vi "DCfgGlbs.vi"() -> ()   [LabVIEW 2011]
panel:
  out "Special[]":i32[](array[numeric])
  in  "Condition":i8[](array[numeric])=[0, 0, 0, 0, 0, 0, 0, 0, 0, 0, 0, 0, 0, 0, 0, 0, 0, 0, 1, 1, 1, 0, 0, 0, 0, 0, 0, 0, -9, 0]
  out "Warning[]":i32[](array[numeric])
  in  "Shutdown[]":i32[](array[numeric])=[5, 9, 11, 12, 20, 21, 22, 28, 29, 30, 31]
  out "Safe[]":i32[](array[numeric])=[0, 6, 8, 13, 14, 15, 16, 27]
  out "Din #":i32
  in  "Din Logic":bool[](array[boolean])=[TRUE, TRUE, TRUE, TRUE, FALSE, FALSE, FALSE, FALSE, TRUE, FALSE, FALSE, FALSE, FALSE, FALSE, FALSE, TRUE, FALSE, TRUE, FALSE, FALSE, FALSE, TRUE, TRUE, TRUE, TRUE, FALSE, FALSE, FALSE, FALSE, FALSE]
  out "Din":string[](array[string])=["Safety/Idle", "LL Routine", "GV Routine", "GC Select", "PANIC Button", "EIS/Pump Overpressure", "TGA Overtemp", "H2 Detector High Alarm", "H2/N2 PD Cell Switch", "H2 Pressure Low", "Pneumatic Pressure Low", "Cabinet Exhaust", "GC Top Doors", "Turbo Fault", "Alkyl H2 Manifold Low", "GV Up (Open)", "GV Down (Open)", "LL Fork Retracted", "Water Alarm - Emore Reactor", "Water Alarm - Ferro", "Water Alarm - F/C", "Emcore Active", "NASA Active", "RF Generator Ready", "RF Power On", "RF Fault", "MDA - GC/LL", "MDA - Gas", "MDA - LL", "MDA - Exhaust"]
  in  "Din Bits":u8[](array[numeric])=[0, 1, 2, 4, 5, 6, 8, 9, 10, 11, 12, 13, 14, 15, 16, 17, 18, 19, 20, 21, 22, 23, 24, 25, 26, 27, 28, 29, 30, 31]
  in  "Din Alarm":u8[](array[numeric])=[0, 0, 0, 0, 1, 6, 7, 9, 0, 8, 10, 11, 12, 13, 14, 0, 0, 0, 15, 16, 17, 0, 0, 0, 0, 18, 2, 3, 4, 5]
  in  "Din Action":u8[](array[numeric])=[1, 0, 0, 0, 2, 1, 1, 2, 0, 2, 2, 1, 1, 1, 1, 0, 0, 0, 2, 2, 2, 0, 0, 0, 0, 1, 2, 2, 2, 2]
  in  "msg":string[](array[string])=["0,No Alarm", "2,PANIC Button Pressed\nSystem Shutdown", "2,MDA High - GC/LL Area\nSystem Shutdown", "2,MDA High - Gas Panel\nSystem Shutdown", "2,MDA High - LL\nSystem Shutdown", "2,MDA High - Exhaust\nSystem  Shutdown", "2,EIS/Pump Overpressure\nSystem  In Safe State", "2,TGA Overtemp\nSystem  In Safe State", "2,H2 Pressure Low\nSystem  In Safe State", "2,H2 Detector High\nSystem In Safe State", "2,Pneumatic Pressure Low\nSystem In Safe State", "2,Cabinet Exhaust\nSystem In Safe State", "1,GC Top Door Open", "1,Turbo Fault", "2,H2 Manifold Low\nSystem  In Safe State", "2,Water - Emcore Reactor\nSystem  In Safe State", "2,Water - Flurrofluidic\nSystem  In Safe State", "2,Water - Flow/GC\nSystem  In Safe State", "2,RF Fault\nSystem  In Safe State", "1,Deviation Alarm", "2,PD _Cell Out Of Temperature\nSystem In Safety State"]
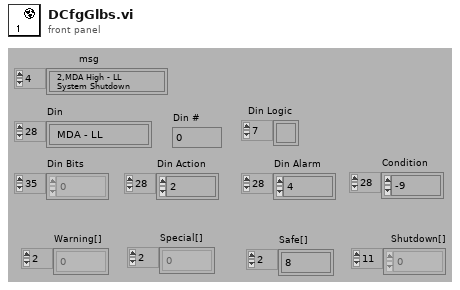
[diagram p1: front panel]
diagram:
